vi "SubVi.Writing data to an ini file.vi"(4 "Input data":T1(array[cluster]), 7 "File with sorted\nand recorded data":path) -> (2 "error":errorcluster)   [LabVIEW 2015]
doc: "Writing data to the ini file, the ini file is created automatically in case of its absence"
uses:
  <vilib>/Utility/config.llb/Write Key (String).vi
  <vilib>/Utility/config.llb/NI_LVConfig.lvlib
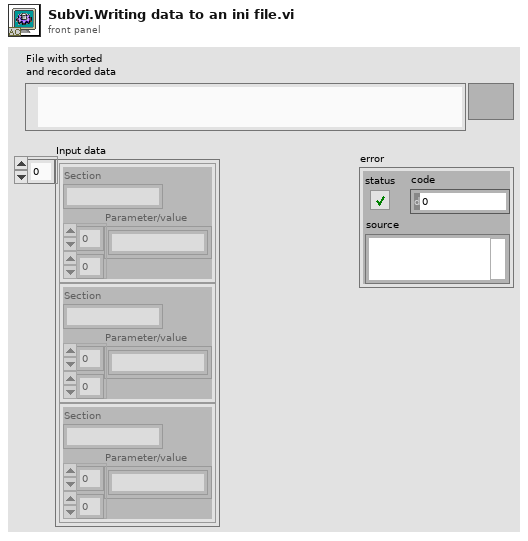
[diagram p1: front panel]
types:
  T1 = cluster{"Section":string, "Parameter/value":string[][]}[]
  T2 = typedef "NI_LVConfig.lvlib/Config Data RefNum.ctl" = refnum<k1>
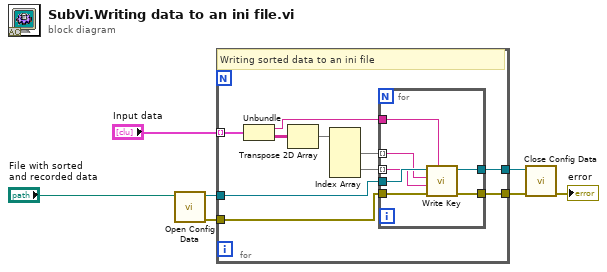
[diagram p0: block diagram]
diagram:
  n1 = call <vilib>:"Open Config Data.vi"("configuration file path"="File with sorted\nand recorded data") -> ("error out"=w3:errorcluster, "refnum"=w2:T2)  [unwired: 8 in, 1 out]
  n2 = for {
    tunnel: "Input data" -> [w17] mode=indexing
    tunnel: w2 -> [w15]
    tunnel: w3 -> [w13]
    tunnel: [w12] -> w4
    tunnel: [w11] -> w5
    # "Writing sorted data to an ini file"
    n3 = Unbundle(w17) -> ("Section"=w16:string, "Parameter/value"=w10:string[][])
    n4 = Transpose 2D Array(2D array=w10) -> (transposed array=w9:string[][])
    n5 = Index Array(array=w9) -> (element #1=w14:string[], element #2=w8:string[])  [unwired: 4 in]
    n6 = for {
      tunnel: w16 -> [w24]
      tunnel: w15 -> [w23]
      tunnel: w14 -> [w21] mode=indexing
      tunnel: w13 -> [w22]
      tunnel: [w19] -> w12
      tunnel: [w20] -> w11
      tunnel: w8 -> [w18] mode=indexing
      n7 = call-poly <vilib>:"Write Key.vi"("section"=w24, "error in (no error)"=w22, "value"=w18, "key"=w21, "refnum"=w23) -> ("error out"=w19:errorcluster, "refnum out"=w20:T2)  [unwired: 4 in, 1 out]
    }
  }
  n8 = call <vilib>:"Close Config Data.vi"("error in (no error)"=w4, "refnum"=w5) -> ("error out"=→"error":errorcluster)  [unwired: 8 in, 1 out]
